vi "TIO RPC Send Heartbeat.vi"(8 "error in (no error)":errorcluster, 11 "TC Connection":T1={"Type"=enum."Serial", "URL"="serial:///dev/cu.usbserial-00000", "TO"=500, "Addr"=0, "Port"=0, "TCP"=refnum, "UDP"=refnum, "Route"=""}) -> (0 "error out":errorcluster, 3 "TC Connection":T1={"Type"=enum."Serial", "URL"="serial:///dev/cu.usbserial-00000", "TO"=500, "Addr"=0, "Port"=0, "TCP"=refnum, "UDP"=refnum, "Route"=""})   [LabVIEW 2020]
uses:
  <instrlib>/tio-labview/TIO Library/TIO SLIP Serial Write.vi
  <instrlib>/tio-labview/TIO Library/TIO Form Packet.vi
  <instrlib>/tio-labview/TIO Library/TIO SLIP Encode.vi
  <instrlib>/tio-labview/TIO Library/TIO Serial Checksum CRC32.vi
panel:
  in  "Boolean":bool
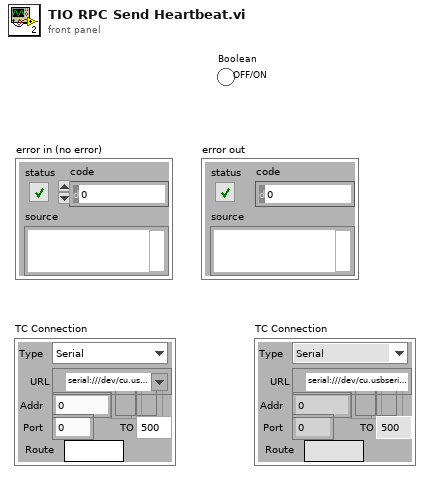
[diagram p1: front panel]
types:
  T1 = cluster{"Type":enum16{"Serial", "TCP", "UDP", "mUDP"}, "URL":refnum<visa-resource-name>, "TO":u32, "Addr":u32, "Port":i32, "TCP":refnum<k5>, "UDP":refnum<k16>, "Route":string}
  T2 = enum8{"Invalid", "Log", "RPC Request", "RPC Reply", "RPC Error", "Heartbeat", "Timebase", "pstream", "dstream", "User"}
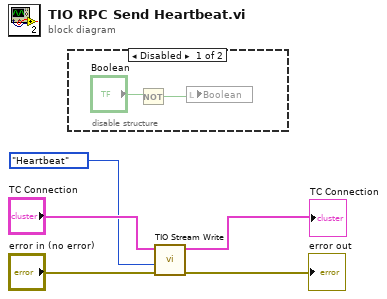
[diagram p0: block diagram]
diagram:
  n1 = disable-structure shown="Disabled" {
    frame Disabled {
      n2 = Not(x="Boolean") -> (.not. x?=w6:bool)
      n3 = local write "Boolean"(w6) -> ()
    }
    frame Enabled {
    }
  }
  n4 = call <instrlib>:"TIO Stream Write.vi"("error in (no error)"="error in (no error)", "Type"=T2."Heartbeat", "TC Connection"="TC Connection") -> ("error out"=→"error out":errorcluster, "TC Connection"=→"TC Connection":T1)  [unwired: 6 in]
